vi "S4GUI_002.vi"(7 "Tab ObsEng":enum32{"Obs", "CCD modes", "Eng"}(tab)) -> ()   [LabVIEW 2018] (continued)
                n3317 = call-dynamic "Read Interface.vi"("error in (no error)"=w7281, "Channel in"=w7284) -> ("error out"=w7292:errorcluster, "Interface.lvclass"=w7293:refnum<class "Interface.lvclass">, "Channel out"=w7310:refnum<class "Channel.lvclass">)  [unwired: 7 in]
                n3318 = call-dynamic "Write Suffix.vi"("error in (no error)"=w7292, "Suffix"=w7300, "Interface in"=w7293) -> ("error out"=w7317:errorcluster, "Interface out"=w7309:refnum<class "Interface.lvclass">)  [unwired: 7 in]
                n3319 = call-dynamic "Write ObsType.vi"("error in (no error)"=w7317, "ObsType"=w7298, "Interface in"=w7309) -> ("error out"=w7316:errorcluster, "Interface out"=w7308:refnum<class "Interface.lvclass">)  [unwired: 7 in]
                n3320 = call-dynamic "Write Object.vi"("error in (no error)"=w7316, "Object"=w7297, "Interface in"=w7308) -> ("error out"=w7315:errorcluster, "Interface out"=w7307:refnum<class "Interface.lvclass">)  [unwired: 7 in]
                n3321 = call-dynamic "Write Comments.vi"("error in (no error)"=w7315, "Comments"=w7299, "Interface in"=w7307) -> ("error out"=w7295:errorcluster, "Interface out"=w7294:refnum<class "Interface.lvclass">)  [unwired: 7 in]
                n3322 = call-dynamic "Write Observer.vi"("error in (no error)"=w7295, "Observer"=w7296, "Interface in"=w7294) -> ("error out"=w7290:errorcluster, "Interface out"=w7291:refnum<class "Interface.lvclass">)  [unwired: 7 in]
                n3323 = call-dynamic "Write Interface.vi"("error in (no error)"=w7290, "Interface.lvclass"=w7291, "Channel in"=w7310) -> ("error out"=w7287:errorcluster, "Channel out"=w7289:refnum<class "Channel.lvclass">)  [unwired: 7 in]
                n3324 = disable-structure shown="Enabled" {
                  disable-tunnel: w7289 -> [w7327 w7329]
                  disable-tunnel: [w7325 w7329] -> w7288
                  disable-tunnel: w7287 -> [w7324 w7328]
                  disable-tunnel: [w7319 w7328] -> w7286
                  frame Disabled {
                    n3325 = call-dynamic "Read State Machine.vi"("error in (no error)"=w7324, "Device in"=w7327) -> ("error out"=w7323:errorcluster, "State Machine.lvclass"=w7321:refnum<class "State Machine.lvclass">, "Device out"=w7326:refnum<class "Channel.lvclass">)  [unwired: 7 in]
                    n3326 = call "Next State.vi"("error in (no error)"=w7323, "New_State"=12, "State Machine in"=w7321) -> ("error out"=w7322:errorcluster, "State Machine out"=w7320:refnum<class "State Machine.lvclass">)  [unwired: 7 in]
                    n3327 = call-dynamic "Write State Machine.vi"("error in (no error)"=w7322, "State Machine.lvclass"=w7320, "Device in"=w7326) -> ("error out"=w7319:errorcluster, "Device out"=w7325:refnum<class "Channel.lvclass">)  [unwired: 7 in]
                  }
                  frame Enabled {
                  }
                }
                n3328 = call-dynamic "Write Channel.vi"("error in (no error)"=w7286, "Channel.lvclass"=w7288, "Acquisition in"=w7305) -> ("error out"=w7303:errorcluster, "Acquisition out"=w7304:refnum<class "Acquisition.lvclass">)  [unwired: 7 in]
                n3329 = call-dynamic "Write AcquisitionA.vi"("error in (no error)"=w7303, "Acquisition.lvclass"=w7304, "S4ACS_GUI in"=w7306) -> ("error out"=w7301:errorcluster, "S4ACS_GUI out"=w7302:refnum<class "S4GUI.lvclass">)  [unwired: 7 in]
              }
              frame #1 {
                # "object"
                # "suffix"
                # "obsType"
                n3330 = call "Read AcquisitionB.vi"("error in (no error)"=w7365, "S4ACS_GUI in"=w7366) -> ("error out"=w7351:errorcluster, "Acquisition.lvclass"=w7352:refnum<class "Acquisition.lvclass">, "S4ACS_GUI out"=w7357:refnum<class "S4GUI.lvclass">)  [unwired: 7 in]
                n3331 = call-dynamic "Read Channel.vi"("error in (no error)"=w7351, "Acquisition in"=w7352) -> ("error out"=w7331:errorcluster, "Channel.lvclass"=w7333:refnum<class "Channel.lvclass">, "Acquisition out"=w7358:refnum<class "Acquisition.lvclass">)  [unwired: 7 in]
                n3332 = local read "Filter2"() -> (w7334:u8)
                n3333 = call-dynamic "Write Filter.vi"("error in (no error)"=w7331, "Filter"=w7334, "Channel in"=w7333) -> ("error out"=w7330:errorcluster, "Channel out"=w7332:refnum<class "Channel.lvclass">)  [unwired: 7 in]
                n3334 = call-dynamic "Read Interface.vi"("error in (no error)"=w7330, "Channel in"=w7332) -> ("error out"=w7339:errorcluster, "Interface.lvclass"=w7340:refnum<class "Interface.lvclass">, "Channel out"=w7353:refnum<class "Channel.lvclass">)  [unwired: 7 in]
                n3335 = call-dynamic "Write Suffix.vi"("error in (no error)"=w7339, "Suffix"=w7362, "Interface in"=w7340) -> ("error out"=w7348:errorcluster, "Interface out"=w7354:refnum<class "Interface.lvclass">)  [unwired: 7 in]
                n3336 = call-dynamic "Write ObsType.vi"("error in (no error)"=w7348, "ObsType"=w7347, "Interface in"=w7354) -> ("error out"=w7349:errorcluster, "Interface out"=w7355:refnum<class "Interface.lvclass">)  [unwired: 7 in]
                n3337 = call-dynamic "Write Object.vi"("error in (no error)"=w7349, "Object"=w7346, "Interface in"=w7355) -> ("error out"=w7350:errorcluster, "Interface out"=w7356:refnum<class "Interface.lvclass">)  [unwired: 7 in]
                n3338 = call-dynamic "Write Comments.vi"("error in (no error)"=w7350, "Comments"=w7361, "Interface in"=w7356) -> ("error out"=w7342:errorcluster, "Interface out"=w7341:refnum<class "Interface.lvclass">)  [unwired: 7 in]
                n3339 = call-dynamic "Write Observer.vi"("error in (no error)"=w7342, "Observer"=w7345, "Interface in"=w7341) -> ("error out"=w7343:errorcluster, "Interface out"=w7344:refnum<class "Interface.lvclass">)  [unwired: 7 in]
                n3340 = call-dynamic "Write Interface.vi"("error in (no error)"=w7343, "Interface.lvclass"=w7344, "Channel in"=w7353) -> ("error out"=w7337:errorcluster, "Channel out"=w7338:refnum<class "Channel.lvclass">)  [unwired: 7 in]
                n3341 = disable-structure shown="Enabled" {
                  disable-tunnel: w7338 -> [w7371 w7378]
                  disable-tunnel: w7337 -> [w7370 w7377]
                  disable-tunnel: [w7368 w7378] -> w7336
                  disable-tunnel: [w7367 w7377] -> w7335
                  frame Disabled {
                    n3342 = call-dynamic "Read State Machine.vi"("error in (no error)"=w7370, "Device in"=w7371) -> ("error out"=w7376:errorcluster, "State Machine.lvclass"=w7374:refnum<class "State Machine.lvclass">, "Device out"=w7369:refnum<class "Channel.lvclass">)  [unwired: 7 in]
                    n3343 = call "Next State.vi"("error in (no error)"=w7376, "New_State"=12, "State Machine in"=w7374) -> ("error out"=w7375:errorcluster, "State Machine out"=w7373:refnum<class "State Machine.lvclass">)  [unwired: 7 in]
                    n3344 = call-dynamic "Write State Machine.vi"("error in (no error)"=w7375, "State Machine.lvclass"=w7373, "Device in"=w7369) -> ("error out"=w7367:errorcluster, "Device out"=w7368:refnum<class "Channel.lvclass">)  [unwired: 7 in]
                  }
                  frame Enabled {
                  }
                }
                n3345 = call-dynamic "Write Channel.vi"("error in (no error)"=w7335, "Channel.lvclass"=w7336, "Acquisition in"=w7358) -> ("error out"=w7360:errorcluster, "Acquisition out"=w7359:refnum<class "Acquisition.lvclass">)  [unwired: 7 in]
                n3346 = call "Write AcquisitionB.vi"("error in (no error)"=w7360, "Acquisition.lvclass"=w7359, "S4ACS_GUI in"=w7357) -> ("error out"=w7363:errorcluster, "S4ACS_GUI out"=w7364:refnum<class "S4GUI.lvclass">)  [unwired: 7 in]
              }
              frame #2 {
                # "object"
                # "suffix"
                # "obsType"
                n3347 = call-dynamic "Read AcquisitionC.vi"("error in (no error)"=w7414, "S4ACS_GUI in"=w7415) -> ("error out"=w7407:errorcluster, "Acquisition.lvclass"=w7406:refnum<class "Acquisition.lvclass">, "S4ACS_GUI out"=w7401:refnum<class "S4GUI.lvclass">)  [unwired: 7 in]
                n3348 = call-dynamic "Read Channel.vi"("error in (no error)"=w7407, "Acquisition in"=w7406) -> ("error out"=w7380:errorcluster, "Channel.lvclass"=w7382:refnum<class "Channel.lvclass">, "Acquisition out"=w7400:refnum<class "Acquisition.lvclass">)  [unwired: 7 in]
                n3349 = local read "Filter3"() -> (w7383:u8)
                n3350 = call-dynamic "Write Filter.vi"("error in (no error)"=w7380, "Filter"=w7383, "Channel in"=w7382) -> ("error out"=w7379:errorcluster, "Channel out"=w7381:refnum<class "Channel.lvclass">)  [unwired: 7 in]
                n3351 = call-dynamic "Read Interface.vi"("error in (no error)"=w7379, "Channel in"=w7381) -> ("error out"=w7392:errorcluster, "Interface.lvclass"=w7393:refnum<class "Interface.lvclass">, "Channel out"=w7405:refnum<class "Channel.lvclass">)  [unwired: 7 in]
                n3352 = call-dynamic "Write Suffix.vi"("error in (no error)"=w7392, "Suffix"=w7411, "Interface in"=w7393) -> ("error out"=w7410:errorcluster, "Interface out"=w7404:refnum<class "Interface.lvclass">)  [unwired: 7 in]
                n3353 = call-dynamic "Write ObsType.vi"("error in (no error)"=w7410, "ObsType"=w7396, "Interface in"=w7404) -> ("error out"=w7409:errorcluster, "Interface out"=w7403:refnum<class "Interface.lvclass">)  [unwired: 7 in]
                n3354 = call-dynamic "Write Object.vi"("error in (no error)"=w7409, "Object"=w7395, "Interface in"=w7403) -> ("error out"=w7408:errorcluster, "Interface out"=w7402:refnum<class "Interface.lvclass">)  [unwired: 7 in]
                n3355 = call-dynamic "Write Comments.vi"("error in (no error)"=w7408, "Comments"=w7397, "Interface in"=w7402) -> ("error out"=w7389:errorcluster, "Interface out"=w7388:refnum<class "Interface.lvclass">)  [unwired: 7 in]
                n3356 = call-dynamic "Write Observer.vi"("error in (no error)"=w7389, "Observer"=w7394, "Interface in"=w7388) -> ("error out"=w7390:errorcluster, "Interface out"=w7391:refnum<class "Interface.lvclass">)  [unwired: 7 in]
                n3357 = call-dynamic "Write Interface.vi"("error in (no error)"=w7390, "Interface.lvclass"=w7391, "Channel in"=w7405) -> ("error out"=w7386:errorcluster, "Channel out"=w7387:refnum<class "Channel.lvclass">)  [unwired: 7 in]
                n3358 = disable-structure shown="Enabled" {
                  disable-tunnel: w7387 -> [w7422 w7427]
                  disable-tunnel: w7386 -> [w7421 w7426]
                  disable-tunnel: [w7419 w7427] -> w7385
                  disable-tunnel: [w7416 w7426] -> w7384
                  frame Disabled {
                    n3359 = call-dynamic "Read State Machine.vi"("error in (no error)"=w7421, "Device in"=w7422) -> ("error out"=w7425:errorcluster, "State Machine.lvclass"=w7418:refnum<class "State Machine.lvclass">, "Device out"=w7420:refnum<class "Channel.lvclass">)  [unwired: 7 in]
                    n3360 = call "Next State.vi"("error in (no error)"=w7425, "New_State"=12, "State Machine in"=w7418) -> ("error out"=w7424:errorcluster, "State Machine out"=w7417:refnum<class "State Machine.lvclass">)  [unwired: 7 in]
                    n3361 = call-dynamic "Write State Machine.vi"("error in (no error)"=w7424, "State Machine.lvclass"=w7417, "Device in"=w7420) -> ("error out"=w7416:errorcluster, "Device out"=w7419:refnum<class "Channel.lvclass">)  [unwired: 7 in]
                  }
                  frame Enabled {
                  }
                }
                n3362 = call-dynamic "Write Channel.vi"("error in (no error)"=w7384, "Channel.lvclass"=w7385, "Acquisition in"=w7400) -> ("error out"=w7398:errorcluster, "Acquisition out"=w7399:refnum<class "Acquisition.lvclass">)  [unwired: 7 in]
                n3363 = call-dynamic "Write AcquisitionC.vi"("error in (no error)"=w7398, "Acquisition.lvclass"=w7399, "S4ACS_GUI in"=w7401) -> ("error out"=w7412:errorcluster, "S4ACS_GUI out"=w7413:refnum<class "S4GUI.lvclass">)  [unwired: 7 in]
              }
              frame #3 {
                # "object"
                # "suffix"
                # "obsType"
                n3364 = call-dynamic "Read AcquisitionD.vi"("error in (no error)"=w7463, "S4ACS_GUI in"=w7464) -> ("error out"=w7456:errorcluster, "Acquisition.lvclass"=w7455:refnum<class "Acquisition.lvclass">, "S4ACS_GUI out"=w7450:refnum<class "S4GUI.lvclass">)  [unwired: 7 in]
                n3365 = call-dynamic "Read Channel.vi"("error in (no error)"=w7456, "Acquisition in"=w7455) -> ("error out"=w7429:errorcluster, "Channel.lvclass"=w7431:refnum<class "Channel.lvclass">, "Acquisition out"=w7449:refnum<class "Acquisition.lvclass">)  [unwired: 7 in]
                n3366 = local read "Filter4"() -> (w7432:u8)
                n3367 = call-dynamic "Write Filter.vi"("error in (no error)"=w7429, "Filter"=w7432, "Channel in"=w7431) -> ("error out"=w7428:errorcluster, "Channel out"=w7430:refnum<class "Channel.lvclass">)  [unwired: 7 in]
                n3368 = call-dynamic "Read Interface.vi"("error in (no error)"=w7428, "Channel in"=w7430) -> ("error out"=w7441:errorcluster, "Interface.lvclass"=w7442:refnum<class "Interface.lvclass">, "Channel out"=w7454:refnum<class "Channel.lvclass">)  [unwired: 7 in]
                n3369 = call-dynamic "Write Suffix.vi"("error in (no error)"=w7441, "Suffix"=w7460, "Interface in"=w7442) -> ("error out"=w7459:errorcluster, "Interface out"=w7453:refnum<class "Interface.lvclass">)  [unwired: 7 in]
                n3370 = call-dynamic "Write ObsType.vi"("error in (no error)"=w7459, "ObsType"=w7445, "Interface in"=w7453) -> ("error out"=w7458:errorcluster, "Interface out"=w7452:refnum<class "Interface.lvclass">)  [unwired: 7 in]
                n3371 = call-dynamic "Write Object.vi"("error in (no error)"=w7458, "Object"=w7444, "Interface in"=w7452) -> ("error out"=w7457:errorcluster, "Interface out"=w7451:refnum<class "Interface.lvclass">)  [unwired: 7 in]
                n3372 = call-dynamic "Write Comments.vi"("error in (no error)"=w7457, "Comments"=w7446, "Interface in"=w7451) -> ("error out"=w7440:errorcluster, "Interface out"=w7439:refnum<class "Interface.lvclass">)  [unwired: 7 in]
                n3373 = call-dynamic "Write Observer.vi"("error in (no error)"=w7440, "Observer"=w7443, "Interface in"=w7439) -> ("error out"=w7438:errorcluster, "Interface out"=w7437:refnum<class "Interface.lvclass">)  [unwired: 7 in]
                n3374 = call-dynamic "Write Interface.vi"("error in (no error)"=w7438, "Interface.lvclass"=w7437, "Channel in"=w7454) -> ("error out"=w7434:errorcluster, "Channel out"=w7436:refnum<class "Channel.lvclass">)  [unwired: 7 in]
                n3375 = disable-structure shown="Enabled" {
                  disable-tunnel: w7436 -> [w7471 w7476]
                  disable-tunnel: [w7469 w7476] -> w7435
                  disable-tunnel: w7434 -> [w7468 w7475]
                  disable-tunnel: [w7467 w7475] -> w7433
                  frame Disabled {
                    n3376 = call-dynamic "Read State Machine.vi"("error in (no error)"=w7468, "Device in"=w7471) -> ("error out"=w7474:errorcluster, "State Machine.lvclass"=w7466:refnum<class "State Machine.lvclass">, "Device out"=w7470:refnum<class "Channel.lvclass">)  [unwired: 7 in]
                    n3377 = call "Next State.vi"("error in (no error)"=w7474, "New_State"=12, "State Machine in"=w7466) -> ("error out"=w7473:errorcluster, "State Machine out"=w7465:refnum<class "State Machine.lvclass">)  [unwired: 7 in]
                    n3378 = call-dynamic "Write State Machine.vi"("error in (no error)"=w7473, "State Machine.lvclass"=w7465, "Device in"=w7470) -> ("error out"=w7467:errorcluster, "Device out"=w7469:refnum<class "Channel.lvclass">)  [unwired: 7 in]
                  }
                  frame Enabled {
                  }
                }
                n3379 = call-dynamic "Write Channel.vi"("error in (no error)"=w7433, "Channel.lvclass"=w7435, "Acquisition in"=w7449) -> ("error out"=w7447:errorcluster, "Acquisition out"=w7448:refnum<class "Acquisition.lvclass">)  [unwired: 7 in]
                n3380 = call-dynamic "Write AcquisitionD.vi"("error in (no error)"=w7447, "Acquisition.lvclass"=w7448, "S4ACS_GUI in"=w7450) -> ("error out"=w7461:errorcluster, "S4ACS_GUI out"=w7462:refnum<class "S4GUI.lvclass">)  [unwired: 7 in]
              }
            }
          }
          frame Enabled {
          }
        }
      }
      event "Observer": Value Change {
        n3381 = event-data() -> ("NewVal"=w7509:string)  [unwired: 1 in, 5 out]
        n3382 = disable-structure shown="Disabled" {
          disable-tunnel: w7512 -> [w7527 w7528]
          disable-tunnel: w7509 -> [w7526 _]
          disable-tunnel: [w7525 w7528] -> w7511
          frame Disabled {
            n3383 = String Length(string=w7526) -> (length=w7524:i32)
            n3384 = Equal To 0?(x=w7524) -> (x = 0?=w7523:bool)
            n3385 = Select(t=u32 16777216, s=w7523, f=u32 16777225) -> (s? t:f=w7521:u32)
            n3386 = property on="Observer" class="Str"(error in=w7527, "Text.BGColor"=w7521) -> (error out=w7525:errorcluster)  [unwired: 1 in, 1 out]
          }
          frame Enabled {
            # "Não se usa mais o texto de fundo\ndo controle \"Observer\""
          }
        }
        n3387 = case shown="False" FALSE {
          tunnel: w7519 -> [w7537 w7735]
          tunnel: w7518 -> [w7536 _]
          tunnel: w7517 -> [w7535 _]
          tunnel: w7516 -> [w7534 _]
          tunnel: w7509 -> [w7533 _]
          tunnel: w7515 -> [w7532 _]
          tunnel: [w7531 w7735] -> w7514
          tunnel: [w7530 w7734] -> w7513
          tunnel: w7511 -> [w7529 w7734]
          frame False {
            n3388 = stacked-sequence {
              seq-local: [w7559 _ _ _] -> [_ w7623 _ _]
              seq-local: [w7558 _ _ _] -> [_ w7622 _ _]
              seq-local: [_ w7621 _ _] -> [_ _ w7672 _]
              seq-local: [_ w7620 _ _] -> [_ _ w7671 _]
              seq-local: [_ _ w7670 _] -> [_ _ _ w7721]
              seq-local: [_ _ w7669 _] -> [_ _ _ w7720]
              tunnel: w7529 -> [w7571 _ _ _]
              tunnel: w7537 -> [w7570 _ _ _]
              tunnel: [_ _ _ w7719] -> w7531
              tunnel: [_ _ _ w7718] -> w7530
              tunnel: w7535 -> [w7557 w7619 w7668 w7717]
              tunnel: w7534 -> [w7556 w7618 w7654 w7703]
              tunnel: w7532 -> [w7555 w7604 w7653 w7702]
              tunnel: w7536 -> [w7554 w7603 w7652 w7701]
              tunnel: w7533 -> [w7553 w7602 w7651 w7700]
              frame #0 {
                # "observer"
                # "comment"
                # "object"
                # "suffix"
                # "obsType"
                n3389 = call-dynamic "Read AcquisitionA.vi"("error in (no error)"=w7571, "S4ACS_GUI in"=w7570) -> ("error out"=w7569:errorcluster, "Acquisition.lvclass"=w7568:refnum<class "Acquisition.lvclass">, "S4ACS_GUI out"=w7563:refnum<class "S4GUI.lvclass">)  [unwired: 7 in]
                n3390 = call-dynamic "Read Channel.vi"("error in (no error)"=w7569, "Acquisition in"=w7568) -> ("error out"=w7539:errorcluster, "Channel.lvclass"=w7542:refnum<class "Channel.lvclass">, "Acquisition out"=w7562:refnum<class "Acquisition.lvclass">)  [unwired: 7 in]
                n3391 = local read "Filter1"() -> (w7540:u8)
                n3392 = call-dynamic "Write Filter.vi"("error in (no error)"=w7539, "Filter"=w7540, "Channel in"=w7542) -> ("error out"=w7538:errorcluster, "Channel out"=w7541:refnum<class "Channel.lvclass">)  [unwired: 7 in]
                n3393 = call-dynamic "Read Interface.vi"("error in (no error)"=w7538, "Channel in"=w7541) -> ("error out"=w7549:errorcluster, "Interface.lvclass"=w7550:refnum<class "Interface.lvclass">, "Channel out"=w7567:refnum<class "Channel.lvclass">)  [unwired: 7 in]
                n3394 = call-dynamic "Write Suffix.vi"("error in (no error)"=w7549, "Suffix"=w7557, "Interface in"=w7550) -> ("error out"=w7574:errorcluster, "Interface out"=w7566:refnum<class "Interface.lvclass">)  [unwired: 7 in]
                n3395 = call-dynamic "Write ObsType.vi"("error in (no error)"=w7574, "ObsType"=w7555, "Interface in"=w7566) -> ("error out"=w7573:errorcluster, "Interface out"=w7565:refnum<class "Interface.lvclass">)  [unwired: 7 in]
                n3396 = call-dynamic "Write Object.vi"("error in (no error)"=w7573, "Object"=w7554, "Interface in"=w7565) -> ("error out"=w7572:errorcluster, "Interface out"=w7564:refnum<class "Interface.lvclass">)  [unwired: 7 in]
                n3397 = call-dynamic "Write Comments.vi"("error in (no error)"=w7572, "Comments"=w7556, "Interface in"=w7564) -> ("error out"=w7552:errorcluster, "Interface out"=w7551:refnum<class "Interface.lvclass">)  [unwired: 7 in]
                n3398 = call-dynamic "Write Observer.vi"("error in (no error)"=w7552, "Observer"=w7553, "Interface in"=w7551) -> ("error out"=w7547:errorcluster, "Interface out"=w7548:refnum<class "Interface.lvclass">)  [unwired: 7 in]
                n3399 = call-dynamic "Write Interface.vi"("error in (no error)"=w7547, "Interface.lvclass"=w7548, "Channel in"=w7567) -> ("error out"=w7544:errorcluster, "Channel out"=w7546:refnum<class "Channel.lvclass">)  [unwired: 7 in]
                n3400 = disable-structure shown="Enabled" {
                  disable-tunnel: w7546 -> [w7584 w7586]
                  disable-tunnel: [w7582 w7586] -> w7545
                  disable-tunnel: w7544 -> [w7581 w7585]
                  disable-tunnel: [w7576 w7585] -> w7543
                  frame Disabled {
                    n3401 = call-dynamic "Read State Machine.vi"("error in (no error)"=w7581, "Device in"=w7584) -> ("error out"=w7580:errorcluster, "State Machine.lvclass"=w7578:refnum<class "State Machine.lvclass">, "Device out"=w7583:refnum<class "Channel.lvclass">)  [unwired: 7 in]
                    n3402 = call "Next State.vi"("error in (no error)"=w7580, "New_State"=12, "State Machine in"=w7578) -> ("error out"=w7579:errorcluster, "State Machine out"=w7577:refnum<class "State Machine.lvclass">)  [unwired: 7 in]
                    n3403 = call-dynamic "Write State Machine.vi"("error in (no error)"=w7579, "State Machine.lvclass"=w7577, "Device in"=w7583) -> ("error out"=w7576:errorcluster, "Device out"=w7582:refnum<class "Channel.lvclass">)  [unwired: 7 in]
                  }
                  frame Enabled {
                  }
                }
                n3404 = call-dynamic "Write Channel.vi"("error in (no error)"=w7543, "Channel.lvclass"=w7545, "Acquisition in"=w7562) -> ("error out"=w7560:errorcluster, "Acquisition out"=w7561:refnum<class "Acquisition.lvclass">)  [unwired: 7 in]
                n3405 = call-dynamic "Write AcquisitionA.vi"("error in (no error)"=w7560, "Acquisition.lvclass"=w7561, "S4ACS_GUI in"=w7563) -> ("error out"=w7558:errorcluster, "S4ACS_GUI out"=w7559:refnum<class "S4GUI.lvclass">)  [unwired: 7 in]
              }
              frame #1 {
                # "object"
                # "suffix"
                # "obsType"
                n3406 = call "Read AcquisitionB.vi"("error in (no error)"=w7622, "S4ACS_GUI in"=w7623) -> ("error out"=w7608:errorcluster, "Acquisition.lvclass"=w7609:refnum<class "Acquisition.lvclass">, "S4ACS_GUI out"=w7614:refnum<class "S4GUI.lvclass">)  [unwired: 7 in]
                n3407 = call-dynamic "Read Channel.vi"("error in (no error)"=w7608, "Acquisition in"=w7609) -> ("error out"=w7588:errorcluster, "Channel.lvclass"=w7590:refnum<class "Channel.lvclass">, "Acquisition out"=w7615:refnum<class "Acquisition.lvclass">)  [unwired: 7 in]
                n3408 = local read "Filter2"() -> (w7591:u8)
                n3409 = call-dynamic "Write Filter.vi"("error in (no error)"=w7588, "Filter"=w7591, "Channel in"=w7590) -> ("error out"=w7587:errorcluster, "Channel out"=w7589:refnum<class "Channel.lvclass">)  [unwired: 7 in]
                n3410 = call-dynamic "Read Interface.vi"("error in (no error)"=w7587, "Channel in"=w7589) -> ("error out"=w7596:errorcluster, "Interface.lvclass"=w7597:refnum<class "Interface.lvclass">, "Channel out"=w7610:refnum<class "Channel.lvclass">)  [unwired: 7 in]
                n3411 = call-dynamic "Write Suffix.vi"("error in (no error)"=w7596, "Suffix"=w7619, "Interface in"=w7597) -> ("error out"=w7605:errorcluster, "Interface out"=w7611:refnum<class "Interface.lvclass">)  [unwired: 7 in]
                n3412 = call-dynamic "Write ObsType.vi"("error in (no error)"=w7605, "ObsType"=w7604, "Interface in"=w7611) -> ("error out"=w7606:errorcluster, "Interface out"=w7612:refnum<class "Interface.lvclass">)  [unwired: 7 in]
                n3413 = call-dynamic "Write Object.vi"("error in (no error)"=w7606, "Object"=w7603, "Interface in"=w7612) -> ("error out"=w7607:errorcluster, "Interface out"=w7613:refnum<class "Interface.lvclass">)  [unwired: 7 in]
                n3414 = call-dynamic "Write Comments.vi"("error in (no error)"=w7607, "Comments"=w7618, "Interface in"=w7613) -> ("error out"=w7599:errorcluster, "Interface out"=w7598:refnum<class "Interface.lvclass">)  [unwired: 7 in]
                n3415 = call-dynamic "Write Observer.vi"("error in (no error)"=w7599, "Observer"=w7602, "Interface in"=w7598) -> ("error out"=w7600:errorcluster, "Interface out"=w7601:refnum<class "Interface.lvclass">)  [unwired: 7 in]
                n3416 = call-dynamic "Write Interface.vi"("error in (no error)"=w7600, "Interface.lvclass"=w7601, "Channel in"=w7610) -> ("error out"=w7594:errorcluster, "Channel out"=w7595:refnum<class "Channel.lvclass">)  [unwired: 7 in]
                n3417 = disable-structure shown="Enabled" {
                  disable-tunnel: w7595 -> [w7628 w7635]
                  disable-tunnel: w7594 -> [w7627 w7634]
                  disable-tunnel: [w7625 w7635] -> w7593
                  disable-tunnel: [w7624 w7634] -> w7592
                  frame Disabled {
                    n3418 = call-dynamic "Read State Machine.vi"("error in (no error)"=w7627, "Device in"=w7628) -> ("error out"=w7633:errorcluster, "State Machine.lvclass"=w7631:refnum<class "State Machine.lvclass">, "Device out"=w7626:refnum<class "Channel.lvclass">)  [unwired: 7 in]
                    n3419 = call "Next State.vi"("error in (no error)"=w7633, "New_State"=12, "State Machine in"=w7631) -> ("error out"=w7632:errorcluster, "State Machine out"=w7630:refnum<class "State Machine.lvclass">)  [unwired: 7 in]
                    n3420 = call-dynamic "Write State Machine.vi"("error in (no error)"=w7632, "State Machine.lvclass"=w7630, "Device in"=w7626) -> ("error out"=w7624:errorcluster, "Device out"=w7625:refnum<class "Channel.lvclass">)  [unwired: 7 in]
                  }
                  frame Enabled {
                  }
                }
                n3421 = call-dynamic "Write Channel.vi"("error in (no error)"=w7592, "Channel.lvclass"=w7593, "Acquisition in"=w7615) -> ("error out"=w7617:errorcluster, "Acquisition out"=w7616:refnum<class "Acquisition.lvclass">)  [unwired: 7 in]
                n3422 = call "Write AcquisitionB.vi"("error in (no error)"=w7617, "Acquisition.lvclass"=w7616, "S4ACS_GUI in"=w7614) -> ("error out"=w7620:errorcluster, "S4ACS_GUI out"=w7621:refnum<class "S4GUI.lvclass">)  [unwired: 7 in]
              }
              frame #2 {
                # "object"
                # "suffix"
                # "obsType"
                n3423 = call-dynamic "Read AcquisitionC.vi"("error in (no error)"=w7671, "S4ACS_GUI in"=w7672) -> ("error out"=w7664:errorcluster, "Acquisition.lvclass"=w7663:refnum<class "Acquisition.lvclass">, "S4ACS_GUI out"=w7658:refnum<class "S4GUI.lvclass">)  [unwired: 7 in]
                n3424 = call-dynamic "Read Channel.vi"("error in (no error)"=w7664, "Acquisition in"=w7663) -> ("error out"=w7637:errorcluster, "Channel.lvclass"=w7639:refnum<class "Channel.lvclass">, "Acquisition out"=w7657:refnum<class "Acquisition.lvclass">)  [unwired: 7 in]
                n3425 = local read "Filter3"() -> (w7640:u8)
                n3426 = call-dynamic "Write Filter.vi"("error in (no error)"=w7637, "Filter"=w7640, "Channel in"=w7639) -> ("error out"=w7636:errorcluster, "Channel out"=w7638:refnum<class "Channel.lvclass">)  [unwired: 7 in]
                n3427 = call-dynamic "Read Interface.vi"("error in (no error)"=w7636, "Channel in"=w7638) -> ("error out"=w7649:errorcluster, "Interface.lvclass"=w7650:refnum<class "Interface.lvclass">, "Channel out"=w7662:refnum<class "Channel.lvclass">)  [unwired: 7 in]
                n3428 = call-dynamic "Write Suffix.vi"("error in (no error)"=w7649, "Suffix"=w7668, "Interface in"=w7650) -> ("error out"=w7667:errorcluster, "Interface out"=w7661:refnum<class "Interface.lvclass">)  [unwired: 7 in]
                n3429 = call-dynamic "Write ObsType.vi"("error in (no error)"=w7667, "ObsType"=w7653, "Interface in"=w7661) -> ("error out"=w7666:errorcluster, "Interface out"=w7660:refnum<class "Interface.lvclass">)  [unwired: 7 in]
                n3430 = call-dynamic "Write Object.vi"("error in (no error)"=w7666, "Object"=w7652, "Interface in"=w7660) -> ("error out"=w7665:errorcluster, "Interface out"=w7659:refnum<class "Interface.lvclass">)  [unwired: 7 in]
                n3431 = call-dynamic "Write Comments.vi"("error in (no error)"=w7665, "Comments"=w7654, "Interface in"=w7659) -> ("error out"=w7646:errorcluster, "Interface out"=w7645:refnum<class "Interface.lvclass">)  [unwired: 7 in]
                n3432 = call-dynamic "Write Observer.vi"("error in (no error)"=w7646, "Observer"=w7651, "Interface in"=w7645) -> ("error out"=w7647:errorcluster, "Interface out"=w7648:refnum<class "Interface.lvclass">)  [unwired: 7 in]
                n3433 = call-dynamic "Write Interface.vi"("error in (no error)"=w7647, "Interface.lvclass"=w7648, "Channel in"=w7662) -> ("error out"=w7643:errorcluster, "Channel out"=w7644:refnum<class "Channel.lvclass">)  [unwired: 7 in]
                n3434 = disable-structure shown="Enabled" {
                  disable-tunnel: w7644 -> [w7679 w7684]
                  disable-tunnel: w7643 -> [w7678 w7683]
                  disable-tunnel: [w7676 w7684] -> w7642
                  disable-tunnel: [w7673 w7683] -> w7641
                  frame Disabled {
                    n3435 = call-dynamic "Read State Machine.vi"("error in (no error)"=w7678, "Device in"=w7679) -> ("error out"=w7682:errorcluster, "State Machine.lvclass"=w7675:refnum<class "State Machine.lvclass">, "Device out"=w7677:refnum<class "Channel.lvclass">)  [unwired: 7 in]
                    n3436 = call "Next State.vi"("error in (no error)"=w7682, "New_State"=12, "State Machine in"=w7675) -> ("error out"=w7681:errorcluster, "State Machine out"=w7674:refnum<class "State Machine.lvclass">)  [unwired: 7 in]
                    n3437 = call-dynamic "Write State Machine.vi"("error in (no error)"=w7681, "State Machine.lvclass"=w7674, "Device in"=w7677) -> ("error out"=w7673:errorcluster, "Device out"=w7676:refnum<class "Channel.lvclass">)  [unwired: 7 in]
                  }
                  frame Enabled {
                  }
                }
                n3438 = call-dynamic "Write Channel.vi"("error in (no error)"=w7641, "Channel.lvclass"=w7642, "Acquisition in"=w7657) -> ("error out"=w7655:errorcluster, "Acquisition out"=w7656:refnum<class "Acquisition.lvclass">)  [unwired: 7 in]
                n3439 = call-dynamic "Write AcquisitionC.vi"("error in (no error)"=w7655, "Acquisition.lvclass"=w7656, "S4ACS_GUI in"=w7658) -> ("error out"=w7669:errorcluster, "S4ACS_GUI out"=w7670:refnum<class "S4GUI.lvclass">)  [unwired: 7 in]
              }
              frame #3 {
                # "object"
                # "suffix"
                # "obsType"
                n3440 = call-dynamic "Read AcquisitionD.vi"("error in (no error)"=w7720, "S4ACS_GUI in"=w7721) -> ("error out"=w7713:errorcluster, "Acquisition.lvclass"=w7712:refnum<class "Acquisition.lvclass">, "S4ACS_GUI out"=w7707:refnum<class "S4GUI.lvclass">)  [unwired: 7 in]
                n3441 = call-dynamic "Read Channel.vi"("error in (no error)"=w7713, "Acquisition in"=w7712) -> ("error out"=w7686:errorcluster, "Channel.lvclass"=w7688:refnum<class "Channel.lvclass">, "Acquisition out"=w7706:refnum<class "Acquisition.lvclass">)  [unwired: 7 in]
                n3442 = local read "Filter4"() -> (w7689:u8)
                n3443 = call-dynamic "Write Filter.vi"("error in (no error)"=w7686, "Filter"=w7689, "Channel in"=w7688) -> ("error out"=w7685:errorcluster, "Channel out"=w7687:refnum<class "Channel.lvclass">)  [unwired: 7 in]
                n3444 = call-dynamic "Read Interface.vi"("error in (no error)"=w7685, "Channel in"=w7687) -> ("error out"=w7698:errorcluster, "Interface.lvclass"=w7699:refnum<class "Interface.lvclass">, "Channel out"=w7711:refnum<class "Channel.lvclass">)  [unwired: 7 in]
                n3445 = call-dynamic "Write Suffix.vi"("error in (no error)"=w7698, "Suffix"=w7717, "Interface in"=w7699) -> ("error out"=w7716:errorcluster, "Interface out"=w7710:refnum<class "Interface.lvclass">)  [unwired: 7 in]
                n3446 = call-dynamic "Write ObsType.vi"("error in (no error)"=w7716, "ObsType"=w7702, "Interface in"=w7710) -> ("error out"=w7715:errorcluster, "Interface out"=w7709:refnum<class "Interface.lvclass">)  [unwired: 7 in]
                n3447 = call-dynamic "Write Object.vi"("error in (no error)"=w7715, "Object"=w7701, "Interface in"=w7709) -> ("error out"=w7714:errorcluster, "Interface out"=w7708:refnum<class "Interface.lvclass">)  [unwired: 7 in]
                n3448 = call-dynamic "Write Comments.vi"("error in (no error)"=w7714, "Comments"=w7703, "Interface in"=w7708) -> ("error out"=w7697:errorcluster, "Interface out"=w7696:refnum<class "Interface.lvclass">)  [unwired: 7 in]
                n3449 = call-dynamic "Write Observer.vi"("error in (no error)"=w7697, "Observer"=w7700, "Interface in"=w7696) -> ("error out"=w7695:errorcluster, "Interface out"=w7694:refnum<class "Interface.lvclass">)  [unwired: 7 in]
                n3450 = call-dynamic "Write Interface.vi"("error in (no error)"=w7695, "Interface.lvclass"=w7694, "Channel in"=w7711) -> ("error out"=w7691:errorcluster, "Channel out"=w7693:refnum<class "Channel.lvclass">)  [unwired: 7 in]
                n3451 = disable-structure shown="Enabled" {
                  disable-tunnel: w7693 -> [w7728 w7733]
                  disable-tunnel: [w7726 w7733] -> w7692
                  disable-tunnel: w7691 -> [w7725 w7732]
                  disable-tunnel: [w7724 w7732] -> w7690
                  frame Disabled {
                    n3452 = call-dynamic "Read State Machine.vi"("error in (no error)"=w7725, "Device in"=w7728) -> ("error out"=w7731:errorcluster, "State Machine.lvclass"=w7723:refnum<class "State Machine.lvclass">, "Device out"=w7727:refnum<class "Channel.lvclass">)  [unwired: 7 in]
                    n3453 = call "Next State.vi"("error in (no error)"=w7731, "New_State"=12, "State Machine in"=w7723) -> ("error out"=w7730:errorcluster, "State Machine out"=w7722:refnum<class "State Machine.lvclass">)  [unwired: 7 in]
                    n3454 = call-dynamic "Write State Machine.vi"("error in (no error)"=w7730, "State Machine.lvclass"=w7722, "Device in"=w7727) -> ("error out"=w7724:errorcluster, "Device out"=w7726:refnum<class "Channel.lvclass">)  [unwired: 7 in]
                  }
                  frame Enabled {
                  }
                }
                n3455 = call-dynamic "Write Channel.vi"("error in (no error)"=w7690, "Channel.lvclass"=w7692, "Acquisition in"=w7706) -> ("error out"=w7704:errorcluster, "Acquisition out"=w7705:refnum<class "Acquisition.lvclass">)  [unwired: 7 in]
                n3456 = call-dynamic "Write AcquisitionD.vi"("error in (no error)"=w7704, "Acquisition.lvclass"=w7705, "S4ACS_GUI in"=w7707) -> ("error out"=w7718:errorcluster, "S4ACS_GUI out"=w7719:refnum<class "S4GUI.lvclass">)  [unwired: 7 in]
              }
            }
          }
          frame True {
          }
        }
      }
      event "Observer": Mouse Enter {
        n3457 = event-data() -> ()  [unwired: 1 in, 4 out]
        n3458 = disable-structure shown="Disabled" {
          disable-tunnel: [w7741 w7744] -> w7737
          disable-tunnel: w7736 -> [w7739 w7744]
          frame Disabled {
            n3459 = property on="Observer" class="Str"() -> ("Value"=w7740:string)  [unwired: 2 in, 2 out]
            n3460 = String Length(string=w7740) -> (length=w7743:i32)
            n3461 = Equal To 0?(x=w7743) -> (x = 0?=w7742:bool)
            n3462 = property on="Observer" class="Str"(error in=w7739, "Caption.Visible"=w7742) -> (error out=w7741:errorcluster)  [unwired: 1 in, 1 out]
          }
          frame Enabled {
            # "Não se usa mais o texto de fundo\ndo controle \"Observer\""
          }
        }
      }
      event "Filter1", "Filter2", "Filter3", "Filter4": Value Change {
        n3463 = event-data() -> ()  [unwired: 1 in, 6 out]
        n3464 = stacked-sequence {
          seq-local: [w7775 _ _ _] -> [_ w7839 _ _]
          seq-local: [w7774 _ _ _] -> [_ w7838 _ _]
          seq-local: [_ w7837 _ _] -> [_ _ w7888 _]
          seq-local: [_ w7836 _ _] -> [_ _ w7887 _]
          seq-local: [_ _ w7886 _] -> [_ _ _ w7937]
          seq-local: [_ _ w7885 _] -> [_ _ _ w7936]
          tunnel: w7752 -> [w7787 _ _ _]
          tunnel: w7753 -> [w7786 _ _ _]
          tunnel: [_ _ _ w7935] -> w7746
          tunnel: [_ _ _ w7934] -> w7745
          tunnel: w7750 -> [w7773 w7835 w7884 w7933]
          tunnel: w7749 -> [w7772 w7834 w7870 w7919]
          tunnel: w7747 -> [w7771 w7820 w7869 w7918]
          tunnel: w7751 -> [w7770 w7819 w7868 w7917]
          tunnel: w7748 -> [w7769 w7818 w7867 w7916]
          frame #0 {
            # "observer"
            # "comment"
            # "object"
            # "suffix"
            # "obsType"
            n3465 = call-dynamic "Read AcquisitionA.vi"("error in (no error)"=w7787, "S4ACS_GUI in"=w7786) -> ("error out"=w7785:errorcluster, "Acquisition.lvclass"=w7784:refnum<class "Acquisition.lvclass">, "S4ACS_GUI out"=w7779:refnum<class "S4GUI.lvclass">)  [unwired: 7 in]
            n3466 = call-dynamic "Read Channel.vi"("error in (no error)"=w7785, "Acquisition in"=w7784) -> ("error out"=w7755:errorcluster, "Channel.lvclass"=w7758:refnum<class "Channel.lvclass">, "Acquisition out"=w7778:refnum<class "Acquisition.lvclass">)  [unwired: 7 in]
            n3467 = local read "Filter1"() -> (w7756:u8)
            n3468 = call-dynamic "Write Filter.vi"("error in (no error)"=w7755, "Filter"=w7756, "Channel in"=w7758) -> ("error out"=w7754:errorcluster, "Channel out"=w7757:refnum<class "Channel.lvclass">)  [unwired: 7 in]
            n3469 = call-dynamic "Read Interface.vi"("error in (no error)"=w7754, "Channel in"=w7757) -> ("error out"=w7765:errorcluster, "Interface.lvclass"=w7766:refnum<class "Interface.lvclass">, "Channel out"=w7783:refnum<class "Channel.lvclass">)  [unwired: 7 in]
            n3470 = call-dynamic "Write Suffix.vi"("error in (no error)"=w7765, "Suffix"=w7773, "Interface in"=w7766) -> ("error out"=w7790:errorcluster, "Interface out"=w7782:refnum<class "Interface.lvclass">)  [unwired: 7 in]
            n3471 = call-dynamic "Write ObsType.vi"("error in (no error)"=w7790, "ObsType"=w7771, "Interface in"=w7782) -> ("error out"=w7789:errorcluster, "Interface out"=w7781:refnum<class "Interface.lvclass">)  [unwired: 7 in]
            n3472 = call-dynamic "Write Object.vi"("error in (no error)"=w7789, "Object"=w7770, "Interface in"=w7781) -> ("error out"=w7788:errorcluster, "Interface out"=w7780:refnum<class "Interface.lvclass">)  [unwired: 7 in]
            n3473 = call-dynamic "Write Comments.vi"("error in (no error)"=w7788, "Comments"=w7772, "Interface in"=w7780) -> ("error out"=w7768:errorcluster, "Interface out"=w7767:refnum<class "Interface.lvclass">)  [unwired: 7 in]
            n3474 = call-dynamic "Write Observer.vi"("error in (no error)"=w7768, "Observer"=w7769, "Interface in"=w7767) -> ("error out"=w7763:errorcluster, "Interface out"=w7764:refnum<class "Interface.lvclass">)  [unwired: 7 in]
            n3475 = call-dynamic "Write Interface.vi"("error in (no error)"=w7763, "Interface.lvclass"=w7764, "Channel in"=w7783) -> ("error out"=w7760:errorcluster, "Channel out"=w7762:refnum<class "Channel.lvclass">)  [unwired: 7 in]
            n3476 = disable-structure shown="Enabled" {
              disable-tunnel: w7762 -> [w7800 w7802]
              disable-tunnel: [w7798 w7802] -> w7761
              disable-tunnel: w7760 -> [w7797 w7801]
              disable-tunnel: [w7792 w7801] -> w7759
              frame Disabled {
                n3477 = call-dynamic "Read State Machine.vi"("error in (no error)"=w7797, "Device in"=w7800) -> ("error out"=w7796:errorcluster, "State Machine.lvclass"=w7794:refnum<class "State Machine.lvclass">, "Device out"=w7799:refnum<class "Channel.lvclass">)  [unwired: 7 in]
                n3478 = call "Next State.vi"("error in (no error)"=w7796, "New_State"=12, "State Machine in"=w7794) -> ("error out"=w7795:errorcluster, "State Machine out"=w7793:refnum<class "State Machine.lvclass">)  [unwired: 7 in]
                n3479 = call-dynamic "Write State Machine.vi"("error in (no error)"=w7795, "State Machine.lvclass"=w7793, "Device in"=w7799) -> ("error out"=w7792:errorcluster, "Device out"=w7798:refnum<class "Channel.lvclass">)  [unwired: 7 in]
              }
              frame Enabled {
              }
            }
            n3480 = call-dynamic "Write Channel.vi"("error in (no error)"=w7759, "Channel.lvclass"=w7761, "Acquisition in"=w7778) -> ("error out"=w7776:errorcluster, "Acquisition out"=w7777:refnum<class "Acquisition.lvclass">)  [unwired: 7 in]
            n3481 = call-dynamic "Write AcquisitionA.vi"("error in (no error)"=w7776, "Acquisition.lvclass"=w7777, "S4ACS_GUI in"=w7779) -> ("error out"=w7774:errorcluster, "S4ACS_GUI out"=w7775:refnum<class "S4GUI.lvclass">)  [unwired: 7 in]
          }
          frame #1 {
            # "object"
            # "suffix"
            # "obsType"
            n3482 = call "Read AcquisitionB.vi"("error in (no error)"=w7838, "S4ACS_GUI in"=w7839) -> ("error out"=w7824:errorcluster, "Acquisition.lvclass"=w7825:refnum<class "Acquisition.lvclass">, "S4ACS_GUI out"=w7830:refnum<class "S4GUI.lvclass">)  [unwired: 7 in]
            n3483 = call-dynamic "Read Channel.vi"("error in (no error)"=w7824, "Acquisition in"=w7825) -> ("error out"=w7804:errorcluster, "Channel.lvclass"=w7806:refnum<class "Channel.lvclass">, "Acquisition out"=w7831:refnum<class "Acquisition.lvclass">)  [unwired: 7 in]
            n3484 = local read "Filter2"() -> (w7807:u8)
            n3485 = call-dynamic "Write Filter.vi"("error in (no error)"=w7804, "Filter"=w7807, "Channel in"=w7806) -> ("error out"=w7803:errorcluster, "Channel out"=w7805:refnum<class "Channel.lvclass">)  [unwired: 7 in]
            n3486 = call-dynamic "Read Interface.vi"("error in (no error)"=w7803, "Channel in"=w7805) -> ("error out"=w7812:errorcluster, "Interface.lvclass"=w7813:refnum<class "Interface.lvclass">, "Channel out"=w7826:refnum<class "Channel.lvclass">)  [unwired: 7 in]
            n3487 = call-dynamic "Write Suffix.vi"("error in (no error)"=w7812, "Suffix"=w7835, "Interface in"=w7813) -> ("error out"=w7821:errorcluster, "Interface out"=w7827:refnum<class "Interface.lvclass">)  [unwired: 7 in]
            n3488 = call-dynamic "Write ObsType.vi"("error in (no error)"=w7821, "ObsType"=w7820, "Interface in"=w7827) -> ("error out"=w7822:errorcluster, "Interface out"=w7828:refnum<class "Interface.lvclass">)  [unwired: 7 in]
            n3489 = call-dynamic "Write Object.vi"("error in (no error)"=w7822, "Object"=w7819, "Interface in"=w7828) -> ("error out"=w7823:errorcluster, "Interface out"=w7829:refnum<class "Interface.lvclass">)  [unwired: 7 in]
            n3490 = call-dynamic "Write Comments.vi"("error in (no error)"=w7823, "Comments"=w7834, "Interface in"=w7829) -> ("error out"=w7815:errorcluster, "Interface out"=w7814:refnum<class "Interface.lvclass">)  [unwired: 7 in]
            n3491 = call-dynamic "Write Observer.vi"("error in (no error)"=w7815, "Observer"=w7818, "Interface in"=w7814) -> ("error out"=w7816:errorcluster, "Interface out"=w7817:refnum<class "Interface.lvclass">)  [unwired: 7 in]
            n3492 = call-dynamic "Write Interface.vi"("error in (no error)"=w7816, "Interface.lvclass"=w7817, "Channel in"=w7826) -> ("error out"=w7810:errorcluster, "Channel out"=w7811:refnum<class "Channel.lvclass">)  [unwired: 7 in]
            n3493 = disable-structure shown="Enabled" {
              disable-tunnel: w7811 -> [w7844 w7851]
              disable-tunnel: w7810 -> [w7843 w7850]
              disable-tunnel: [w7841 w7851] -> w7809
              disable-tunnel: [w7840 w7850] -> w7808
              frame Disabled {
                n3494 = call-dynamic "Read State Machine.vi"("error in (no error)"=w7843, "Device in"=w7844) -> ("error out"=w7849:errorcluster, "State Machine.lvclass"=w7847:refnum<class "State Machine.lvclass">, "Device out"=w7842:refnum<class "Channel.lvclass">)  [unwired: 7 in]
                n3495 = call "Next State.vi"("error in (no error)"=w7849, "New_State"=12, "State Machine in"=w7847) -> ("error out"=w7848:errorcluster, "State Machine out"=w7846:refnum<class "State Machine.lvclass">)  [unwired: 7 in]
                n3496 = call-dynamic "Write State Machine.vi"("error in (no error)"=w7848, "State Machine.lvclass"=w7846, "Device in"=w7842) -> ("error out"=w7840:errorcluster, "Device out"=w7841:refnum<class "Channel.lvclass">)  [unwired: 7 in]
              }
              frame Enabled {
              }
            }
            n3497 = call-dynamic "Write Channel.vi"("error in (no error)"=w7808, "Channel.lvclass"=w7809, "Acquisition in"=w7831) -> ("error out"=w7833:errorcluster, "Acquisition out"=w7832:refnum<class "Acquisition.lvclass">)  [unwired: 7 in]
            n3498 = call "Write AcquisitionB.vi"("error in (no error)"=w7833, "Acquisition.lvclass"=w7832, "S4ACS_GUI in"=w7830) -> ("error out"=w7836:errorcluster, "S4ACS_GUI out"=w7837:refnum<class "S4GUI.lvclass">)  [unwired: 7 in]
          }
          frame #2 {
            # "object"
            # "suffix"
            # "obsType"
            n3499 = call-dynamic "Read AcquisitionC.vi"("error in (no error)"=w7887, "S4ACS_GUI in"=w7888) -> ("error out"=w7880:errorcluster, "Acquisition.lvclass"=w7879:refnum<class "Acquisition.lvclass">, "S4ACS_GUI out"=w7874:refnum<class "S4GUI.lvclass">)  [unwired: 7 in]
            n3500 = call-dynamic "Read Channel.vi"("error in (no error)"=w7880, "Acquisition in"=w7879) -> ("error out"=w7854:errorcluster, "Channel.lvclass"=w7856:refnum<class "Channel.lvclass">, "Acquisition out"=w7873:refnum<class "Acquisition.lvclass">)  [unwired: 7 in]
            n3501 = local read "Filter3"() -> (w7857:u8)
            n3502 = call-dynamic "Write Filter.vi"("error in (no error)"=w7854, "Filter"=w7857, "Channel in"=w7856) -> ("error out"=w7853:errorcluster, "Channel out"=w7855:refnum<class "Channel.lvclass">)  [unwired: 7 in]
            n3503 = call-dynamic "Read Interface.vi"("error in (no error)"=w7853, "Channel in"=w7855) -> ("error out"=w7865:errorcluster, "Interface.lvclass"=w7866:refnum<class "Interface.lvclass">, "Channel out"=w7878:refnum<class "Channel.lvclass">)  [unwired: 7 in]
            n3504 = call-dynamic "Write Suffix.vi"("error in (no error)"=w7865, "Suffix"=w7884, "Interface in"=w7866) -> ("error out"=w7883:errorcluster, "Interface out"=w7877:refnum<class "Interface.lvclass">)  [unwired: 7 in]
            n3505 = call-dynamic "Write ObsType.vi"("error in (no error)"=w7883, "ObsType"=w7869, "Interface in"=w7877) -> ("error out"=w7882:errorcluster, "Interface out"=w7876:refnum<class "Interface.lvclass">)  [unwired: 7 in]
            n3506 = call-dynamic "Write Object.vi"("error in (no error)"=w7882, "Object"=w7868, "Interface in"=w7876) -> ("error out"=w7881:errorcluster, "Interface out"=w7875:refnum<class "Interface.lvclass">)  [unwired: 7 in]
            n3507 = call-dynamic "Write Comments.vi"("error in (no error)"=w7881, "Comments"=w7870, "Interface in"=w7875) -> ("error out"=w7862:errorcluster, "Interface out"=w7861:refnum<class "Interface.lvclass">)  [unwired: 7 in]
            n3508 = call-dynamic "Write Observer.vi"("error in (no error)"=w7862, "Observer"=w7867, "Interface in"=w7861) -> ("error out"=w7863:errorcluster, "Interface out"=w7864:refnum<class "Interface.lvclass">)  [unwired: 7 in]
            n3509 = call-dynamic "Write Interface.vi"("error in (no error)"=w7863, "Interface.lvclass"=w7864, "Channel in"=w7878) -> ("error out"=w7859:errorcluster, "Channel out"=w7860:refnum<class "Channel.lvclass">)  [unwired: 7 in]
            n3510 = disable-structure shown="Enabled" {
              disable-tunnel: w7860 -> [w7895 w7900]
              disable-tunnel: w7859 -> [w7894 w7899]
              disable-tunnel: [w7889 w7899] -> w7858
              disable-tunnel: [w7892 w7900] -> w7852
              frame Disabled {
                n3511 = call-dynamic "Read State Machine.vi"("error in (no error)"=w7894, "Device in"=w7895) -> ("error out"=w7898:errorcluster, "State Machine.lvclass"=w7891:refnum<class "State Machine.lvclass">, "Device out"=w7893:refnum<class "Channel.lvclass">)  [unwired: 7 in]
                n3512 = call "Next State.vi"("error in (no error)"=w7898, "New_State"=12, "State Machine in"=w7891) -> ("error out"=w7897:errorcluster, "State Machine out"=w7890:refnum<class "State Machine.lvclass">)  [unwired: 7 in]
                n3513 = call-dynamic "Write State Machine.vi"("error in (no error)"=w7897, "State Machine.lvclass"=w7890, "Device in"=w7893) -> ("error out"=w7889:errorcluster, "Device out"=w7892:refnum<class "Channel.lvclass">)  [unwired: 7 in]
              }
              frame Enabled {
              }
            }
            n3514 = call-dynamic "Write Channel.vi"("error in (no error)"=w7858, "Channel.lvclass"=w7852, "Acquisition in"=w7873) -> ("error out"=w7871:errorcluster, "Acquisition out"=w7872:refnum<class "Acquisition.lvclass">)  [unwired: 7 in]
            n3515 = call-dynamic "Write AcquisitionC.vi"("error in (no error)"=w7871, "Acquisition.lvclass"=w7872, "S4ACS_GUI in"=w7874) -> ("error out"=w7885:errorcluster, "S4ACS_GUI out"=w7886:refnum<class "S4GUI.lvclass">)  [unwired: 7 in]
          }
          frame #3 {
            # "object"
            # "suffix"
            # "obsType"
            n3516 = call-dynamic "Read AcquisitionD.vi"("error in (no error)"=w7936, "S4ACS_GUI in"=w7937) -> ("error out"=w7929:errorcluster, "Acquisition.lvclass"=w7928:refnum<class "Acquisition.lvclass">, "S4ACS_GUI out"=w7923:refnum<class "S4GUI.lvclass">)  [unwired: 7 in]
            n3517 = call-dynamic "Read Channel.vi"("error in (no error)"=w7929, "Acquisition in"=w7928) -> ("error out"=w7902:errorcluster, "Channel.lvclass"=w7904:refnum<class "Channel.lvclass">, "Acquisition out"=w7922:refnum<class "Acquisition.lvclass">)  [unwired: 7 in]
            n3518 = local read "Filter4"() -> (w7905:u8)
            n3519 = call-dynamic "Write Filter.vi"("error in (no error)"=w7902, "Filter"=w7905, "Channel in"=w7904) -> ("error out"=w7901:errorcluster, "Channel out"=w7903:refnum<class "Channel.lvclass">)  [unwired: 7 in]
            n3520 = call-dynamic "Read Interface.vi"("error in (no error)"=w7901, "Channel in"=w7903) -> ("error out"=w7914:errorcluster, "Interface.lvclass"=w7915:refnum<class "Interface.lvclass">, "Channel out"=w7927:refnum<class "Channel.lvclass">)  [unwired: 7 in]
            n3521 = call-dynamic "Write Suffix.vi"("error in (no error)"=w7914, "Suffix"=w7933, "Interface in"=w7915) -> ("error out"=w7932:errorcluster, "Interface out"=w7926:refnum<class "Interface.lvclass">)  [unwired: 7 in]
            n3522 = call-dynamic "Write ObsType.vi"("error in (no error)"=w7932, "ObsType"=w7918, "Interface in"=w7926) -> ("error out"=w7931:errorcluster, "Interface out"=w7925:refnum<class "Interface.lvclass">)  [unwired: 7 in]
            n3523 = call-dynamic "Write Object.vi"("error in (no error)"=w7931, "Object"=w7917, "Interface in"=w7925) -> ("error out"=w7930:errorcluster, "Interface out"=w7924:refnum<class "Interface.lvclass">)  [unwired: 7 in]
            n3524 = call-dynamic "Write Comments.vi"("error in (no error)"=w7930, "Comments"=w7919, "Interface in"=w7924) -> ("error out"=w7913:errorcluster, "Interface out"=w7912:refnum<class "Interface.lvclass">)  [unwired: 7 in]
            n3525 = call-dynamic "Write Observer.vi"("error in (no error)"=w7913, "Observer"=w7916, "Interface in"=w7912) -> ("error out"=w7911:errorcluster, "Interface out"=w7910:refnum<class "Interface.lvclass">)  [unwired: 7 in]
            n3526 = call-dynamic "Write Interface.vi"("error in (no error)"=w7911, "Interface.lvclass"=w7910, "Channel in"=w7927) -> ("error out"=w7907:errorcluster, "Channel out"=w7909:refnum<class "Channel.lvclass">)  [unwired: 7 in]
            n3527 = disable-structure shown="Enabled" {
              disable-tunnel: w7909 -> [w7944 w7949]
